vi "Write Versions.vi"(8 "error in (no error)":errorcluster, 10 "Versions":refnum<class "Package Version.lvclass">[](array[class]), 11 "Package in":refnum<class "Package.lvclass">) -> (0 "error out":errorcluster, 3 "Package out":refnum<class "Package.lvclass">)   [LabVIEW 2020, in "Packages.lvlib" / "Package.lvclass"]
uses:
  Package.lvclass
  Package Version_class/Package Version.lvclass
  Package.lvclass/Package.ctl
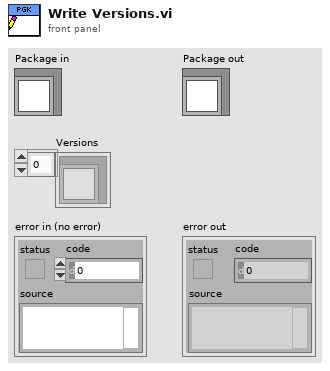
[diagram p1: front panel]
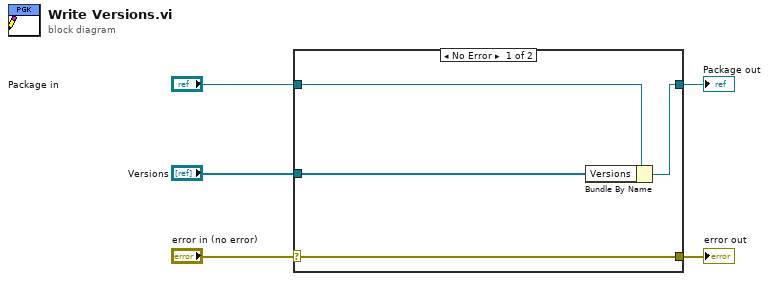
[diagram p0: block diagram]
diagram:
  n1 = case shown="No Error" "error in (no error)" {
    selector: "error in (no error)" -> [w9 w10]
    tunnel: [w9 w10] -> w4
    tunnel: [w7 w11] -> w2
    tunnel: "Package in" -> [w8 w11]
    tunnel: "Versions" -> [w6 _]
    frame No Error {
      n2 = Bundle By Name(cluster=w8, "Versions"=w6) -> (w7:refnum<class "Package.lvclass">)
    }
    frame Error {
    }
  }
  "error out" <- w4
  "Package out" <- w2
